vi "BundleErrors.vi"(1 "base path":path) -> (0 "AllErrors":path)   [LabVIEW 2012]
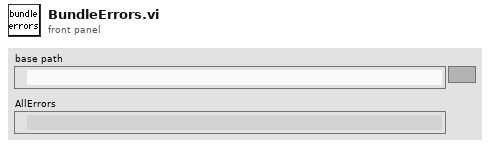
[diagram p1: front panel]
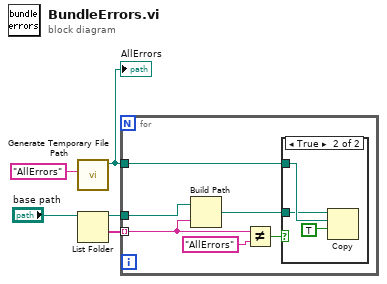
[diagram p0: block diagram]
diagram:
  n1 = call <vilib>:"Generate Temporary File Path.vi"("Temporary File Extension (tmp)"="AllErrors" ("name or relative path")) -> ("Unique Temporary File Path"=w1:path)  [unwired: 9 in, 1 out]
  "AllErrors" <- w1
  n2 = List Folder(path="base path") -> (path out=w4:path, folder names=w3:string[])  [unwired: 3 in, 2 out]
  n3 = for {
    tunnel: w1 -> [w11]
    tunnel: w4 -> [w10]
    tunnel: w3 -> [w7] mode=indexing
    n4 = Build Path(base path=w10, name or relative path=w7) -> (appended path=w9:path)
    n5 = Not Equal?(x=w7, y="AllErrors") -> (x != y?=w8:bool)
    n6 = case shown="True" w8 {
      tunnel: w11 -> [_ w14]
      tunnel: w9 -> [_ w13]
      frame False {
      }
      frame True {
        n7 = Copy(9:TRUE ("overwrite (F)"), 10:w14, 11:w13) -> ()  [unwired: 2 in, 3 out]
      }
    }
  }
